vi "LEBITplc.ProcPeriodic.vi"(0 "i ref in":refnum<vi>, 3 "ms timeout (10000)":i32=10000, 5 "error in (no error)":errorcluster) -> (14 "i ref out":refnum<vi>, 17 "timed out":bool, 19 "error out":errorcluster)   [LabVIEW 2014, in "LEBITplc.lvlib"]
doc: "This method serves to periodically do things like reading values from the HW. Methods that should be executed periodically should be called from THIS methode. Add code here."
uses:
  LEBITplc.lvlib
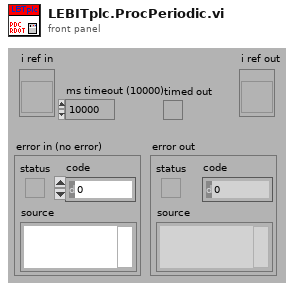
[diagram p1: front panel]
types:
  T1 = typedef "LEBITplc.lvlib/LEBITplc.i attribute.ctl" = cluster{"LLFLocation":string, "SetFileLocation":string, "nickNames":string[], "setValuePLCServiceID":i32[], "GUIServiceID":i32[], "monValuePLC":string[], "SetValueServiceID":i32[], "MonValueServiceID":i32[], "SetValue":dbl[][], "SetValueMin":dbl[], "SetValueMax":dbl[], "SetValueInfoServiceID":i32[], "GUINames":string[], "ListOfBases":string[], "Scale":dbl[], "Offset":dbl[], "setValuePLC":string[], "BaseName":string[], "ScaleServiceID":i32[], "OffsetServiceID":i32[], "AllPLCValues":string[], "CondSpecialArray":string[][], "CondSpecialIndex":i32[], "CondSpecialMonValue":dbl[], "RecentlyChanged":i32[], "SetFileLocationID":i32, "Dependent-Monitors":string[][], "LastLoadedFiles":string[], "IonGuideCalibLocation":string, "Monitor Dependent":string[], "Special":string[], "PLC?":bool[], "Start Date":string, "ListOfBasesServiceID":i32, "SETRA VISA resource":refnum<visa-resource-name>}
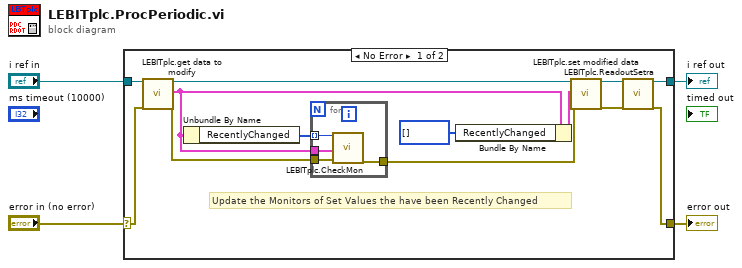
[diagram p0: block diagram]
diagram:
  n1 = case shown="No Error" "error in (no error)" {
    selector: "error in (no error)" -> [w11 w22]
    tunnel: "i ref in" -> [w17 w23]
    tunnel: [w7 w23] -> w2
    tunnel: [w5 w22] -> w1
    frame No Error {
      # "Update the Monitors of Set Values the have been Recently Changed"
      n2 = call "LEBITplc.get data to modify.vi"("i ref in"=w17, "error in (no error)"=w11) -> ("i ref out"=w15:refnum<vi>, "i attribute"=w12:T1, "error out"=w10:errorcluster)  [unwired: 14 in, 1 out]
      n3 = Unbundle By Name(w12) -> ("RecentlyChanged"=w16:i32[])
      n4 = for {
        tunnel: w16 -> [w21] mode=indexing
        tunnel: w12 -> [w20]
        tunnel: w10 -> [w19]
        tunnel: [w18] -> w9
        n5 = call "LEBITplc.CheckMon.vi"("index of element"=w21, "i attribute in"=w20, "error in"=w19) -> ("error IO"=w18:errorcluster)  [unwired: 16 in]
      }
      n6 = Bundle By Name(cluster=w12, "RecentlyChanged"=i32[] []) -> (w14:T1)
      n7 = call "LEBITplc.set modified data.vi"("i ref in"=w15, "i attribute"=w14, "error in (no error)"=w9) -> ("i ref out"=w8:refnum<vi>, "error out"=w6:errorcluster)  [unwired: 15 in]
      n8 = call "LEBITplc.ReadoutSetra.vi"("i ref in"=w8, "error in"=w6) -> ("i ref out"=w7:refnum<vi>, "error IO"=w5:errorcluster)  [unwired: 16 in]
    }
    frame Error {
    }
  }
  "error out" <- w1
  "i ref out" <- w2
